vi "Run.vi"(8 "error in (no error)":errorcluster, 11 "SiemensDigitalEnergyMeter in":refnum<class "SiemensDigitalEnergyMeter.lvclass">) -> (0 "error out":errorcluster, 1 "DataValid":bool, 2 "clSensorData":T1, 3 "SiemensDigitalEnergyMeter out":refnum<class "SiemensDigitalEnergyMeter.lvclass">)   [LabVIEW 2018, in "SensorPlugins.lvlib" / "SiemensDigitalEnergyMeter.lvclass"]
doc: "This VI retrieves measurements from the Siemens Digital Energy Meter."
uses:
  SiemensDigitalEnergyMeter.lvclass
  SensorShared/clSensorData.ctl
  SensorShared/SensorVisulization.ctl
  <vilib>/NI/Modbus Library/API/Master/Modbus Master.lvclass
  SensorShared/SensorShared.lvlib
panel:
  out "Execution Time (ms)":u32
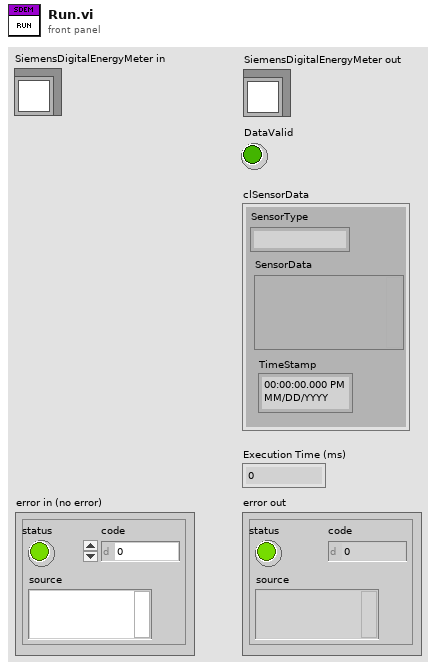
[diagram p1: front panel]
types:
  T1 = typedef "SensorShared.lvlib/clSensorData.ctl" = cluster{"SensorType":string, "SensorData":variant, "TimeStamp":timestamp}
  T2 = typedef "SensorShared.lvlib/SensorVisulization.ctl" = cluster{"Array of Waveforms":waveform(dbl)[], "Array of Strings ":string[], "LightTower":cluster{"Red":bool, "Amber":bool, "Green":bool, "Audio":bool}}
  T3 = typedef "SensorPlugins.lvlib/SiemensDigitalEnergyMeter.lvclass/CommunicationControls.ctl" = refnum<class "Modbus Master.lvclass">[]
  T4 = typedef "SensorPlugins.lvlib/SiemensDigitalEnergyMeter.lvclass/SiemensDigitalEnergyMeterControls.ctl" = cluster{"Measurement(s)":u16[], "Configuration Commands":string, "Use Measurement Commands Text Box?":bool, "Measurement Commands":string, "Connected?":bool, "Serial Number":string, "IP Address":string, "Port (502)":u16, "Unit ID":u8, "Serial Type":enum16{"RTU", "ASCII"}, "Using TCP?":bool, "VISA Resource Name":string}[]
  T5 = typedef "SensorPlugins.lvlib/SiemensDigitalEnergyMeter.lvclass/MeasurementControls.ctl" = cluster{"Measurement RefreshTime (ms)":u32, "Measurement Name":string}
  T6 = cluster{"Measurement(s)":u16[], "Configuration Commands":string, "Use Measurement Commands Text Box?":bool, "Measurement Commands":string, "Connected?":bool, "Serial Number":string, "IP Address":string, "Port (502)":u16, "Unit ID":u8, "Serial Type":enum16{"RTU", "ASCII"}, "Using TCP?":bool, "VISA Resource Name":string}
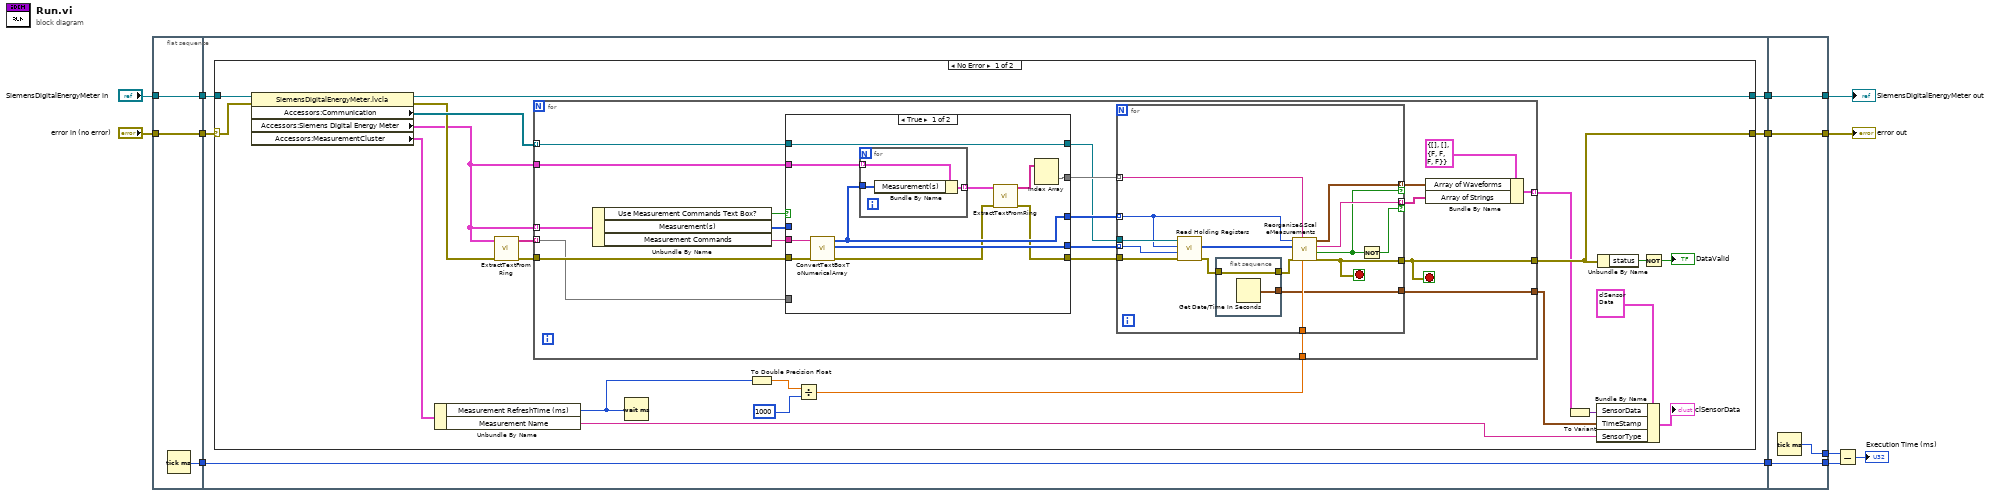
[diagram p0: block diagram]
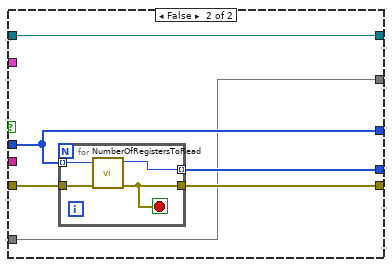
[diagram p2: hidden frame]
diagram:
  n1 = flat-sequence {
    tunnel: "SiemensDigitalEnergyMeter in" -> [w15]
    tunnel: "error in (no error)" -> [w16]
    tunnel: [w16] -> w9
    tunnel: [w15] -> w8
    tunnel: [w14] -> w7
    tunnel: w9 -> [w21]
    tunnel: w8 -> [w20]
    tunnel: [w19] -> w6
    tunnel: [w18] -> w5
    tunnel: w7 -> [w17]
    tunnel: [w17] -> w4
    tunnel: [w109] -> w10
    tunnel: [w110] -> w11
    tunnel: w4 -> [w107]
    tunnel: w5 -> [w109]
    tunnel: w6 -> [w110]
    tunnel: [w108] -> w2
    tunnel: [w107] -> w1
    frame #0 {
      n2 = Tick Count (ms)() -> (millisecond timer value=w14:u32)
    }
    frame #1 {
      n3 = case shown="No Error" w21 {
        selector: w21 -> [w42 w106]
        tunnel: w20 -> [w43 w105]
        tunnel: [w30 w106] -> w18
        tunnel: [w41 w105] -> w19
        frame No Error {
          n4 = property class="SiemensDigitalEnergyMeter.lvcla"(reference=w43, error in=w42) -> (reference out=w41:refnum<class "SiemensDigitalEnergyMeter.lvclass">, error out=w36:errorcluster, "Accessors:Communication"=w40:T3, "Accessors:Siemens Digital Energy Meter"=w33:T4, "Accessors:MeasurementCluster"=w29:T5)
          n5 = Unbundle By Name(w29) -> ("Measurement RefreshTime (ms)"=w25:u32, "Measurement Name"=w23:string)
          n6 = call "ExtractTextFromRing.vi"("error in (no error)"=w36, "Siemens Digital Energy Meter"=w33) -> ("error out"=w35:errorcluster, "MeasurementTypeStrings"=w34:string[][])  [unwired: 8 in]
          n7 = Wait (ms)(milliseconds to wait=w25) -> ()  [unwired: 1 out]
          n8 = To Double Precision Float(number=w25) -> (double precision float=w26:dbl)
          n9 = Divide(x=w26, y=u32 1000) -> (x/y=w24:dbl)
          n10 = for {
            tunnel: w33 -> [w55] mode=indexing
            tunnel: w35 -> [w60]
            tunnel: [w59] -> w30
            tunnel: w40 -> [w48] mode=indexing
            tunnel: w34 -> [w53] mode=indexing
            tunnel: w33 -> [w54]
            tunnel: [w49] -> w28 mode=indexing
            tunnel: w24 -> [w45]
            tunnel: [w44] -> w22
            stop <- w59 stop-if-true
            n11 = Unbundle By Name(w55) -> ("Use Measurement Commands Text Box?"=w63:bool, "Measurement(s)"=w62:u16[], "Measurement Commands"=w61:string)
            n12 = case shown="True" w63 {
              tunnel: [w65 w82] -> w56
              tunnel: w62 -> [_ w81]
              tunnel: w61 -> [w73 _]
              tunnel: w60 -> [w74 w83]
              tunnel: [w71 w81] -> w58
              tunnel: [w72 w80] -> w57
              tunnel: w54 -> [w70 _]
              tunnel: w53 -> [_ w79]
              tunnel: [w66 w79] -> w52
              tunnel: w48 -> [w64 w78]
              tunnel: [w64 w78] -> w47
              frame True {
                n13 = call "ConvertTextBoxToNumericalArray.vi"("Error In"=w74, "Configuration Commands"=w73) -> ("Error Out"=w68:errorcluster, "Register Value"=w72:u16[], "Register"=w71:u16[])  [unwired: 7 in]
                n14 = for {
                  tunnel: w71 -> [w77]
                  tunnel: w70 -> [w76] mode=indexing
                  tunnel: [w75] -> w69 mode=indexing
                  n15 = Bundle By Name(cluster=w76, "Measurement(s)"=w77) -> (w75:T6)
                }
                n16 = call "ExtractTextFromRing.vi"("error in (no error)"=w68, "Siemens Digital Energy Meter"=w69) -> ("error out"=w65:errorcluster, "MeasurementTypeStrings"=w67:string[][])  [unwired: 8 in]
                n17 = Index Array(array=w67) -> (element=w66:string[])  [unwired: 2 in]
              }
              frame False {
                n18 = for {
                  tunnel: [w86] -> w80 mode=indexing
                  tunnel: w81 -> [w85] mode=indexing
                  tunnel: w83 -> [w87]
                  tunnel: [w84] -> w82
                  stop <- w84 stop-if-true
                  n19 = call "NumberOfRegistersToRead.vi"("Error In"=w87, "Measurement TextRing"=w85) -> ("Error Out"=w84:errorcluster, "Numer of Registers"=w86:u16)  [unwired: 8 in]
                }
              }
            }
            n20 = for {
              tunnel: [w102] -> w59
              tunnel: [w101] -> w50 mode=indexing if=w98
              tunnel: [w100] -> w51 mode=indexing if=w99
              tunnel: w56 -> [w95]
              tunnel: w47 -> [w94]
              tunnel: w58 -> [w93] mode=indexing
              tunnel: w57 -> [w92] mode=indexing
              tunnel: w52 -> [w97] mode=indexing
              tunnel: w45 -> [w91]
              tunnel: [w88] -> w44
              stop <- w102 stop-if-true
              n21 = call-dynamic "Read Holding Registers.vi"("error in"=w95, "number of inputs"=w92, "starting address"=w93, "Modbus master in"=w94) -> ("error out"=w90:errorcluster, "register values"=w96:u16[])  [unwired: 5 in, 1 out]
              n22 = flat-sequence {
                tunnel: w90 -> [w104]
                tunnel: [w104] -> w89
                tunnel: [w103] -> w88
                frame #0 {
                  n23 = Get Date/Time In Seconds() -> (seconds since 1Jan1904=w103:timestamp)
                }
              }
              n24 = call "Reorganize&ScaleMeasurements.vi"("dt"=w91, "MeasurementType"=w97, "Error In"=w89, "Register Values"=w96, "Measurement TextRing"=w93) -> ("Error Out"=w102:errorcluster, "Numerical Information"=w98:bool, "String"=w100:string, "output waveform"=w101:waveform(dbl))  [unwired: 3 in]
              n25 = Not(x=w98) -> (.not. x?=w99:bool)
            }
            n26 = Bundle By Name(cluster=T2 {"Array of Waveforms"=[], "Array of Strings "=[], "LightTower"={"Red"=FALSE, "Amber"=FALSE, "Green"=FALSE, "Audio"=FALSE}} ("SiemensDEMMeasurements 2"), "Array of Waveforms"=w50, "Array of Strings"=w51) -> (w49:T2)
          }
          n27 = To Variant(anything=w28) -> (Variant=w37:variant)
          n28 = Bundle By Name(cluster=T1 {"SensorType"="", "SensorData"=variant, "TimeStamp"=timestamp(0 s since 1904-01-01)} ("clSensorData"), "SensorData"=w37, "TimeStamp"=w22, "SensorType"=w23) -> (→"clSensorData":T1)
          n29 = Unbundle By Name(w30) -> ("status"=w31:bool)
          n30 = Not(x=w31) -> (.not. x?=→"DataValid":bool)
        }
        frame Error {
        }
      }
    }
    frame #2 {
      n31 = Tick Count (ms)() -> (millisecond timer value=w108:u32)
    }
  }
  n32 = Subtract(x=w2, y=w1) -> (x-y=→"Execution Time (ms)":u32)
  "error out" <- w10
  "SiemensDigitalEnergyMeter out" <- w11
